vi "SetRoomWalls.vi"(8 "error in (no error)":errorcluster, 9 "DirectionsList":T1[](array[typedef]), 10 "Room":refnum<class "Room.lvclass">, 11 "MazeGame in":refnum<class "MazeGame.lvclass">) -> (0 "error out":errorcluster, 3 "MazeGame out":refnum<class "MazeGame.lvclass">)   [LabVIEW 2020, in "FactoryMethod.lvlib" / "ParameterizedFactoryMethod.lvlib" / "MazeGame.lvclass"]
uses:
  MazeGame.lvclass
  GoFcommonClasses/Direction.ctl
  GoFcommonClasses/ConcreteMazeSite/Room/Room.lvclass
  GoFcommonClasses/ConcreteMazeSite/Wall/Wall.lvclass
  E:/Francesco/GitHub/Design-Patterns-GoF_-_NI-LV/Creational/GoFcommonClasses/MazeSite/MazeSite.lvclass
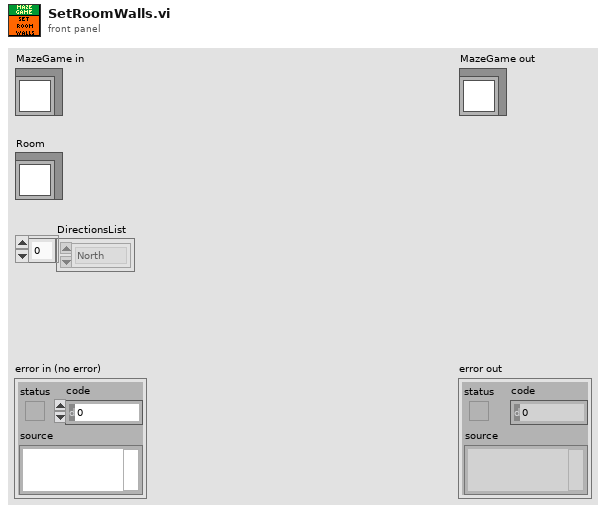
[diagram p1: front panel]
types:
  T1 = typedef "Direction.ctl" = enum32{"North", "South", "East", "West"}
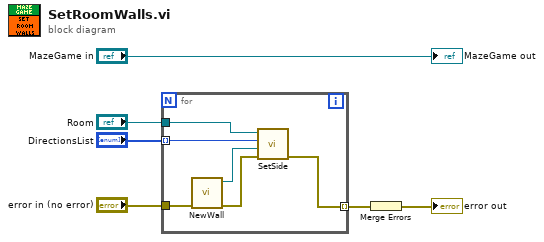
[diagram p0: block diagram]
diagram:
  n1 = for {
    tunnel: "DirectionsList" -> [w10] mode=indexing
    tunnel: "Room" -> [w12]
    tunnel: [w11] -> w3 mode=indexing
    tunnel: "error in (no error)" -> [w8]
    n2 = call "NewWall.vi"("error in (no error)"=w8) -> ("error out"=w7:errorcluster, "Wall"=w9:refnum<class "Wall.lvclass">)  [unwired: 9 in]
    n3 = call "SetSide.vi"("error in (no error)"=w7, "MazeSite"=w9, "Direction"=w10, "Room in"=w12) -> ("error out"=w11:errorcluster)  [unwired: 6 in, 1 out]
  }
  n4 = Merge Errors(w3) -> (→"error out":errorcluster)
  "MazeGame out" <- "MazeGame in"
